vi "Display_Module.vi"(7 "Command":T3, 8 "error in (no error)":errorcluster, 9 "Data":variant, 10 "Data Type":T2, 11 "user event out":T1) -> (0 "error out":errorcluster)   [LabVIEW 2017]
uses:
  Display_Command Control.ctl
  Data Type.ctl
  User Event Reference.ctl
  User Event Data.ctl
panel:
  # "Input Data"
  # "Local Data"
  # "Output Data"
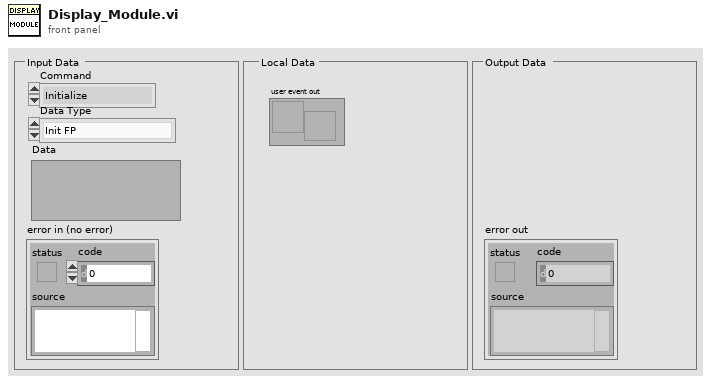
[diagram p1: front panel]
types:
  T1 = typedef "User Event Reference.ctl" = refnum<user-event>
  T2 = typedef "Data Type.ctl" = enum16{"Init FP", "En/Dis FP Ctls", "Update FP", "Upd Status", "Upd Seq"}
  T3 = typedef "Display_Command Control.ctl" = enum16{"Initialize", "Generate Event", "Shutdown"}
  T4 = typedef "User Event Data.ctl" = cluster{"Data Type":T2, "Data":variant}
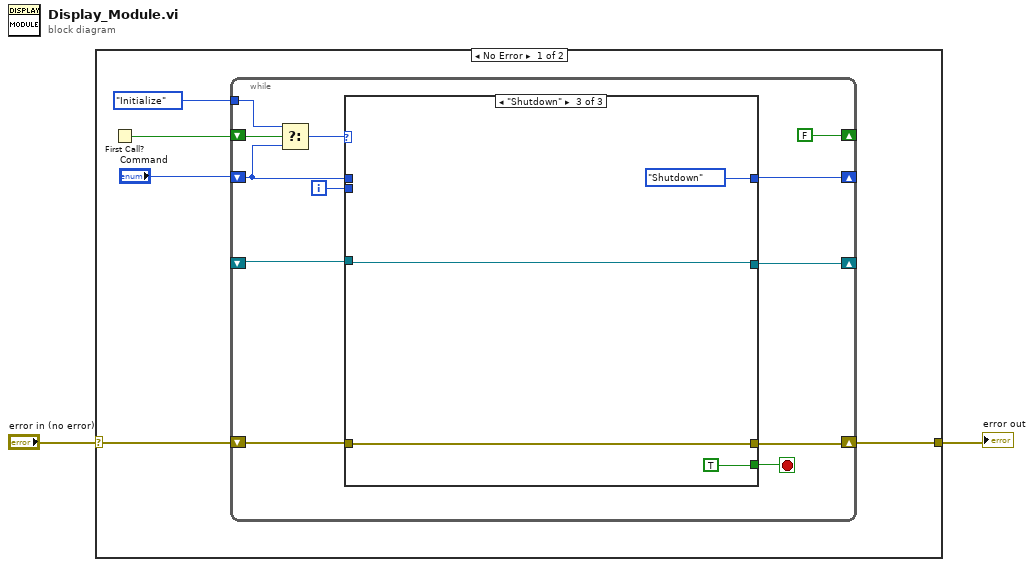
[diagram p0: block diagram]
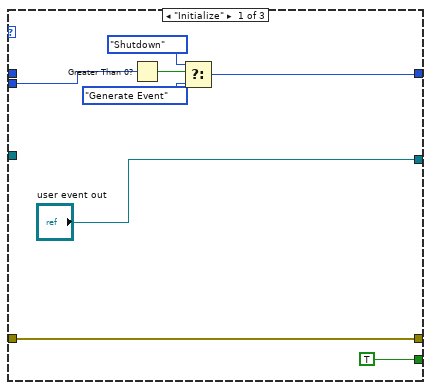
[diagram p2: hidden frame]
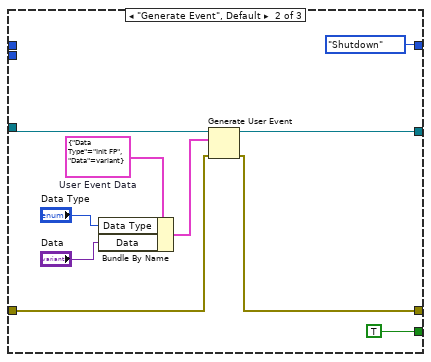
[diagram p3: hidden frame]
diagram:
  n1 = case shown="No Error" "error in (no error)" {
    selector: "error in (no error)" -> [w6 w42]
    tunnel: [w5 w42] -> w1
    frame No Error {
      n2 = First Call?() -> (First Call?: T/F=w7:bool)
      n3 = while {
        shift-right: [w11] -> _
        shift-left: "Command" -> [w12]
        shift-right: [w14] -> w5
        shift-left: w6 -> [w15]
        shift-right: [FALSE ("First Call?: T/F")] -> _
        shift-left: w7 -> [w19]
        tunnel: Display_Command_Control."Initialize" ("Command") -> [w18]
        shift-right: [w9] -> _
        shift-left: _ -> [w8]
        i -> [w10]
        stop <- w16 stop-if-true
        n4 = Select(t=w18, s=w19, f=w12) -> (s? t:f=w17:T3)
        n5 = case shown="\"Shutdown\"" w17 {
          tunnel: [TRUE TRUE TRUE] -> w16
          tunnel: w15 -> [w26 w30 w40]
          tunnel: [w26 w29 w40] -> w14
          tunnel: w12 -> [_ _ _]
          tunnel: [w25 Display_Command_Control."Shutdown" ("t") Display_Command_Control."Shutdown"] -> w11
          tunnel: w10 -> [w23 _ _]
          tunnel: ["user event out" w34 w38] -> w9
          tunnel: w8 -> [_ w35 w38]
          frame "Initialize" {
            n6 = Greater Than 0?(x=w23) -> (x > 0?=w22:bool)
            n7 = Select(t=Display_Command_Control."Shutdown", s=w22, f=Display_Command_Control."Generate Event" ("t")) -> (s? t:f=w25:T3)
          }
          frame "Generate Event", Default {
            w28 = T4 {"Data Type"=enum."Init FP", "Data"=variant}  # User Event Data
            n8 = Bundle By Name(cluster=w28, "Data Type"="Data Type", "Data"="Data") -> (w31:T4)
            n9 = Generate User Event(user event=w35, event data cluster=w31, error in=w30) -> (user event out=w34:T1, error out=w29:errorcluster)  [unwired: 1 in]
          }
          frame "Shutdown" {
          }
        }
      }
    }
    frame Error {
    }
  }
  "error out" <- w1
